vi "Edgertronic-dir_listing.vi"(3 "error in (no error)":errorcluster, 5 "URL":string="192.168.1.101") -> (0 "error out":errorcluster, 1 "Directory Listing:":T1, 2 "Movies":string[](array[string]))   [LabVIEW 2015]
doc: "This VI returns the list of files in the active storage video directory."
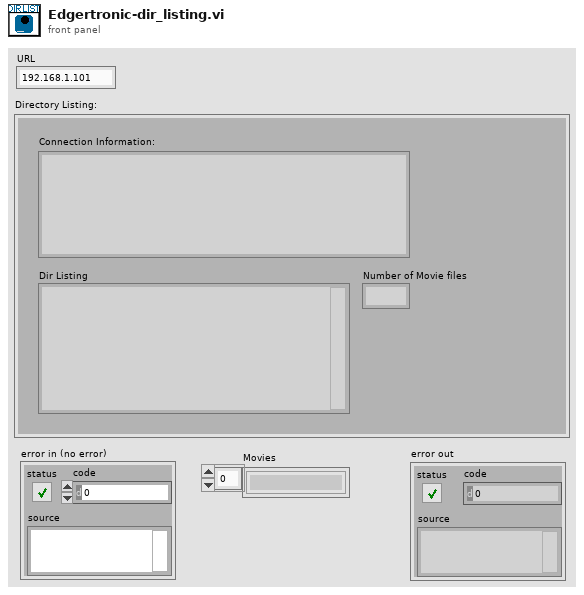
[diagram p1: front panel]
types:
  T1 = cluster{"Connection Information:":string, "Dir Listing":string, "Number of Movie files":string}
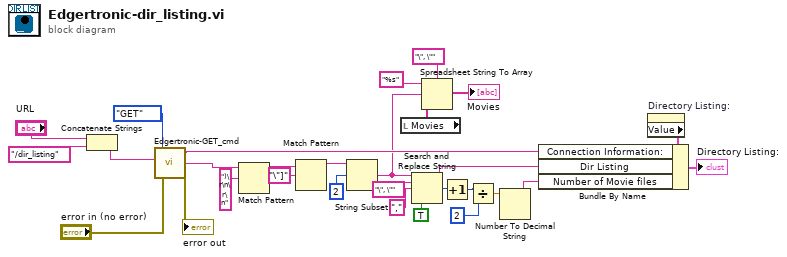
[diagram p0: block diagram]
diagram:
  n1 = Concatenate Strings("URL", "/dir_listing" ("GET Cmd")) -> (w2:string)
  n2 = call "Edgertronic-GET_cmd.vi"("error in (no error)"="error in (no error)", "URL"=w2, "Type"=enum16{"GET", "POST"}."GET") -> ("error out"=→"error out":errorcluster, "data"=w12:string, "Connection Info"=w13:string)  [unwired: 1 in]
  n3 = Match Pattern(string=w12, regular expression=")\r\n\r\n") -> (before substring=w16:string)  [unwired: 1 in, 3 out]
  n4 = Match Pattern(string=w16, regular expression="\"]") -> (before substring=w28:string)  [unwired: 1 in, 3 out]
  n5 = String Subset(string=w28, offset (0)=2) -> (substring=w8:string)  [unwired: 1 in]
  n6 = local read "Movies"() -> (w5:string[])
  n7 = Search and Replace String(replace all?=TRUE ("replace all? (F)"), input string=w8, search string="\", \"" ("regular expression (\"\")"), replace string="," ("replace string (\"\")")) -> (result string=w10:string, number of replacements=w23:i32)  [unwired: 4 in, 2 out]
  n8 = Spreadsheet String To Array(delimiter (Tab)="\", \"" ("regular expression (\"\")"), format string="%s", spreadsheet string=w8, array type (2D Dbl)=w5) -> (array=→"Movies":string[])
  n9 = Increment(x=w23) -> (x+1=w21:i32)
  n10 = Divide(x=w21, y=2) -> (x/y=w18:dbl)
  n11 = Number To Decimal String(number=w18) -> (decimal integer string=w17:string)  [unwired: 1 in]
  n12 = property on="Directory Listing:" class="Clust (strict)"() -> ("Value"=w15:T1)  [unwired: 2 in, 2 out]
  n13 = Bundle By Name(cluster=w15, "Connection Information:"=w13, "Dir Listing"=w10, "Number of Movie files"=w17) -> (→"Directory Listing:":T1)
